vi "Is Actor Class or Interface.vi"(6 "Validation":T1, 8 "error in (no error)":errorcluster, 10 "Target in":refnum<vi>, 11 "LVClass Library in":refnum<vi>) -> (0 "error out":errorcluster, 1 "is actor?":bool, 2 "TargetItem out":refnum<vi>, 4 "is actor interface?":bool)   [LabVIEW 2020, in "Message Maker.lvlib"]
uses:
  Message Maker.lvlib
  AFPP Shared/Validation Mode.ctl
  AFPP Shared/AFPP Shared.lvlib
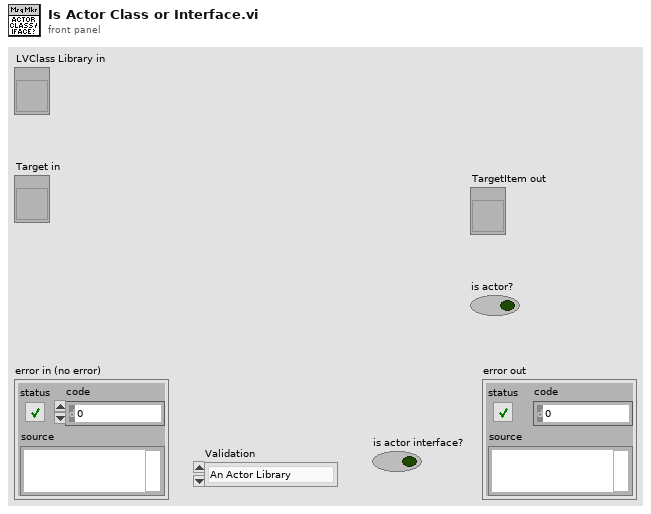
[diagram p1: front panel]
types:
  T1 = typedef "AFPP Shared.lvlib/Validation Mode.ctl" = enum16{"An Actor Library", "A Target Tag"}
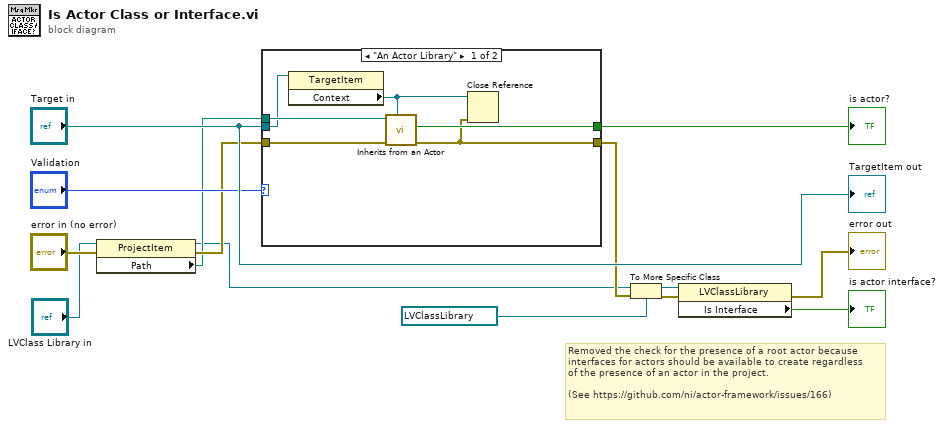
[diagram p0: block diagram]
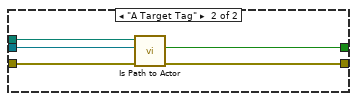
[diagram p2: hidden frame]
diagram:
  # "Removed the check for the presence of a root actor because\ninterfaces for actors should be available to create regardless\nof the presence of an actor in the project.\n\n(See https://github.com/ni/actor-framework/issues/166)"
  n1 = property class="ProjectItem"(reference="LVClass Library in", error in="error in (no error)") -> (reference out=w2:refnum<vi>, error out=w5:errorcluster, "Path"=w4:path)
  n2 = case shown="\"An Actor Library\"" "Validation" {
    tunnel: w5 -> [w19 w25]
    tunnel: [w16 w24] -> w7
    tunnel: w4 -> [w20 w23]
    tunnel: [w18 w22] -> w11
    tunnel: "Target in" -> [w17 w21]
    frame "An Actor Library" {
      n3 = property class="TargetItem"(reference=w17) -> ("Context"=w15:refnum<vi>)  [unwired: 1 in, 2 out]
      n4 = call "Inherits from an Actor.vi"("App Reference (this app)"=w15, "error in (no error)"=w19, "Path"=w20) -> ("error out"=w16:errorcluster, "Is Path to Actor?"=w18:bool)  [unwired: 6 in, 1 out]
      n5 = Close Reference(reference=w15, error in (no error)=w16) -> ()  [unwired: 1 out]
    }
    frame "A Target Tag" {
      n6 = call "Is Path to Actor.vi"("error in (no error)"=w25, "Target"=w21, "Path"=w23) -> ("error out"=w24:errorcluster, "Is Path to Actor?"=w22:bool)  [unwired: 6 in, 1 out]
    }
  }
  "is actor?" <- w11
  n7 = To More Specific Class(target class=refnum<vi> refnum ("LVClassLibrary in"), reference=w2, error in=w7) -> (specific class reference=w9:refnum<vi>, error out=w8:errorcluster)
  n8 = property class="LVClassLibrary"(reference=w9, error in=w8) -> (error out=→"error out":errorcluster, "Is Interface"=→"is actor interface?":bool)  [unwired: 1 out]
  "TargetItem out" <- "Target in"
